vi "what dont like.vi"() -> ()   [LabVIEW 2017]
uses:
  what.ctl
  <vilib>/myRIO/Instrument Drivers/Onboard IO/DIO/typedefs/DIO Reference.ctl
  <vilib>/myRIO/Common/Instrument Driver Framework/Utilities/typedefs/myRIO Generic Hardware Reference.ctl
  <vilib>/myRIO/Common/Instrument Driver Framework/Utilities/typedefs/Hardware Version Enum.ctl
  <vilib>/myRIO/Common/Instrument Driver Framework/Utilities/typedefs/myRIO v1.0 Reference.ctl
  <vilib>/myRIO/Common/Instrument Driver Framework/Utilities/typedefs/Generic FPGA Reference.ctl
  <vilib>/myRIO/Common/Instrument Driver Framework/myRIO v1.0/DIO/typedefs/DIO Channels List.ctl
  <vilib>/myRIO/Common/Instrument Driver Framework/myRIO v1.0/DIO/typedefs/DIO Channels Enum.ctl
  <vilib>/userdefined/High Color/nirio_resource_hc.ctl
  <vilib>/myRIO/Common/Instrument Driver Framework/Utilities/vis/Is FPGA Ref Available.vi
  <vilib>/myRIO/Common/Instrument Driver Framework/myRIO v1.0/DIO/vis/myRIO v1.1 Open DIO.vi
  <vilib>/myRIO/Instrument Drivers/Onboard IO/DIO/vis/Read.vi
  <vilib>/myRIO/Common/Instrument Driver Framework/Utilities/vis/Validate Channels.vi
  <vilib>/myRIO/Common/Instrument Driver Framework/myRIO v1.0/DIO/vis/myRIO v1.0 Reserve DIO.vi
  <vilib>/myRIO/Common/Instrument Driver Framework/myRIO v1.0/Resource Manager/vis/myRIO v1.0 Reserve Channel List.vi
  <vilib>/myRIO/Common/Instrument Driver Framework/myRIO v1.0/DIO/vis/myRIO v1.0 Build MUX Configuration DIO.vi
  <vilib>/myRIO/Common/Instrument Driver Framework/myRIO v1.0/Resource Manager/vis/myRIO v1.0 Reserve Channel.vi
  <vilib>/myRIO/Common/Instrument Driver Framework/myRIO v1.0/Resource Manager/vis/myRIO v1.0 Unreserve Channel.vi
  <vilib>/myRIO/Common/Instrument Driver Framework/myRIO v1.0/Resource Manager/vis/myRIO v1.0 Create Configuration List.vi
  <vilib>/myRIO/Common/Instrument Driver Framework/myRIO v1.0/Resource Manager/vis/myRIO v1.0 Build Mutex Name.vi
  <vilib>/Utility/VariantDataType/GetNumericInfo.vi
  <vilib>/Utility/error.llb/Error Cluster From Error Code.vi
  <vilib>/myRIO/Common/Instrument Driver Framework/myRIO v1.0/myRIO v1.1 Open.vi
  <vilib>/myRIO/Common/Instrument Driver Framework/Utilities/vis/IO Manager.vi
  <vilib>/myRIO/Common/Instrument Driver Framework/Utilities/vis/Configuration Manager.vi
  <vilib>/myRIO/Common/Instrument Driver Framework/myRIO v1.0/Resource Manager/vis/myRIO v1.0 Configure IO.vi
  <vilib>/myRIO/Common/Instrument Driver Framework/myRIO v1.0/myRIO v1.0 Close.vi
  <vilib>/myRIO/Common/Instrument Driver Framework/myRIO v1.0/DIO/vis/myRIO v1.0 Read DIO.vi
  <vilib>/myRIO/Express VI/Onboard IO/DI/DI Express VI.xnode
  <vilib>/myRIO/Instrument Drivers/Onboard IO/DIO/vis/myRIO DIO Open.xnode
  <vilib>/myRIO/Instrument Drivers/Onboard IO/DIO/DIO.lvlib
panel:
  out "index of element":i32
  in  "Stop":bool
  out "Counter Value":dbl
  in  "stop":bool
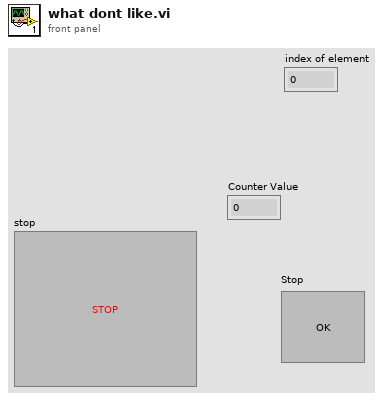
[diagram p1: front panel]
types:
  T1 = typedef "what.ctl" = enum16{"Initialize", "Floor 1", "Floor 2", "Floor 3", "GO!", "Stop!", "Wait for User Input"}
  T2 = typedef "DIO.lvlib/DIO Reference.ctl" = cluster{"myRIO Reference":T3, "DIO Channels List":T7}
  T3 = typedef "myRIO Generic Hardware Reference.ctl" = cluster{"myRIO Model":T4, "myRIO Hardware Reference":T5}
  T4 = typedef "Hardware Version Enum.ctl" = enum16{"Unknown", "myRIO-1900", "myRIO-1950", "roboRIO", "NI ELVIS RIO CM"}
  T5 = typedef "myRIO v1.0 Reference.ctl" = cluster{"Generic FPGA Reference":T6, "Allow multiple opens":bool}
  T6 = typedef "Generic FPGA Reference.ctl" = refnum<k20>
  T7 = typedef "DIO Channels List.ctl" = T8[]
  T8 = typedef "DIO Channels Enum.ctl" = enum16{"Not Connected", "C/DIO0", "C/DIO1", "C/DIO2", "C/DIO3", "C/DIO4", "C/DIO5", "C/DIO6", "C/DIO7", "A/DIO0", "A/DIO1", "A/DIO2", "A/DIO3", "A/DIO4", "A/DIO5", "A/DIO6", "A/DIO7", "A/DIO8", "A/DIO9", "A/DIO10", "A/DIO11", "A/DIO12", "A/DIO13", "A/DIO14", "A/DIO15", "B/DIO0", "B/DIO1", "B/DIO2", "B/DIO3", "B/DIO4", "B/DIO5", "B/DIO6", "B/DIO7", "B/DIO8", "B/DIO9", "B/DIO10", "B/DIO11", "B/DIO12", "B/DIO13", "B/DIO14", "B/DIO15", "LED0", "LED1", "LED2", "LED3", "Button0", "DIO/DIO0", "DIO/DIO1", "DIO/DIO2", "DIO/DIO3", "DIO/DIO4", "DIO/DIO5", "DIO/DIO6", "DIO/DIO7", "DIO/DIO8", "DIO/DIO9", "SPI/CS0", "SPI/CS1", "SPI/CS2", "SPI/CS3", "LED RADIO (Green)", "LED RADIO (Red)", "LED COMM (Green)", "LED COMM (Red)", "LED MODE (Green)", "LED MODE (Red)"}
  T9 = typedef "nirio_resource_hc.ctl" = tag
  T10 = enum16{"off", "flash", "top", "middle", "bottom"}
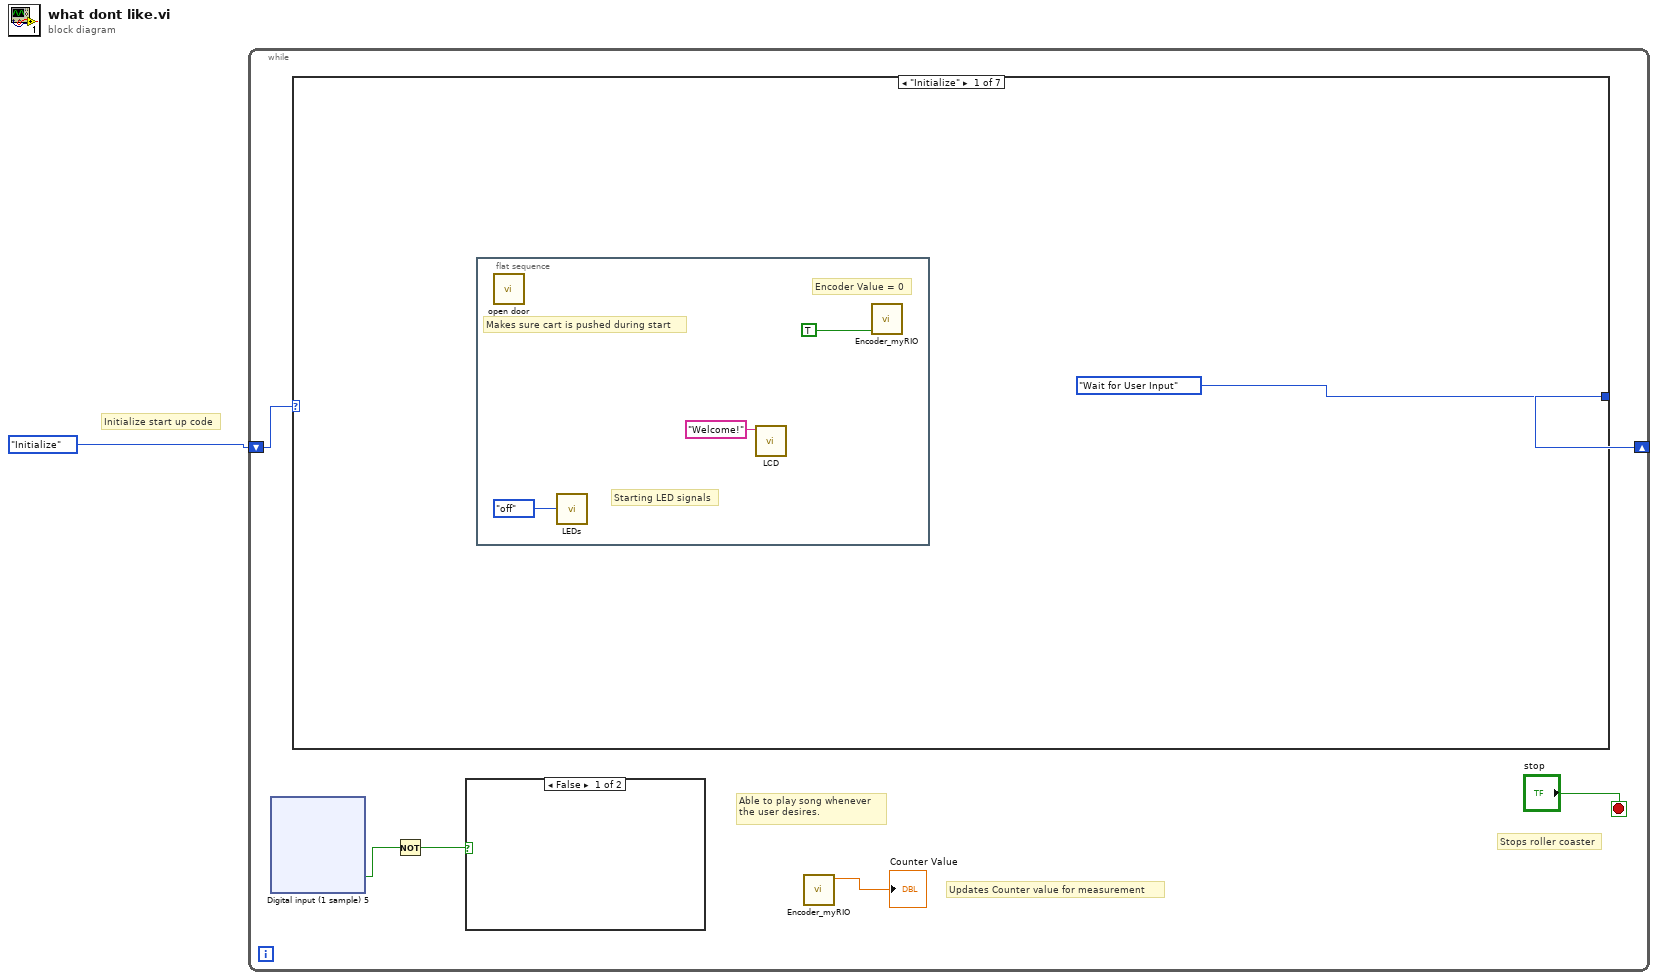
[diagram p0: block diagram]
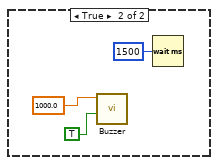
[diagram p2: hidden frame]
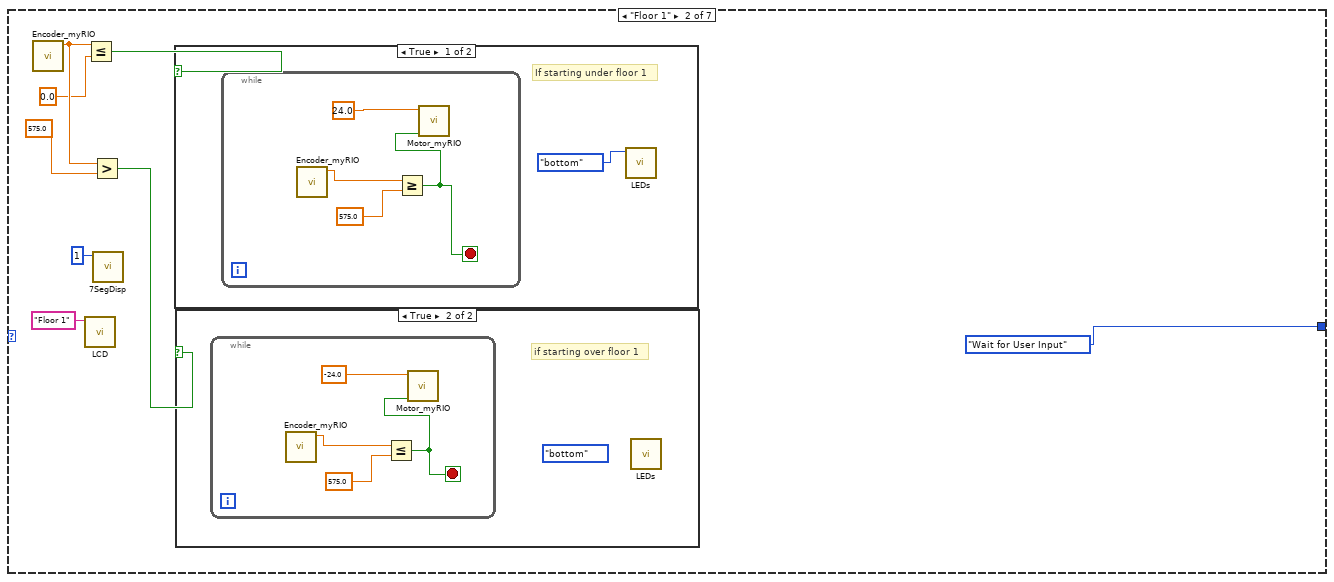
[diagram p3: hidden frame]
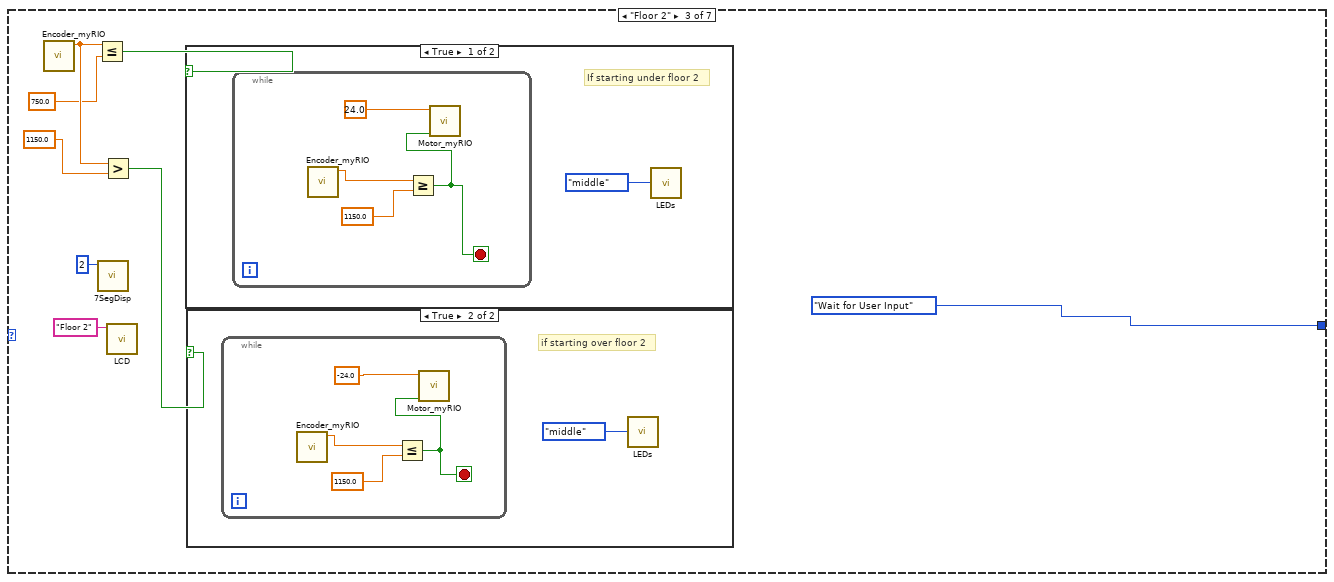
[diagram p6: hidden frame]
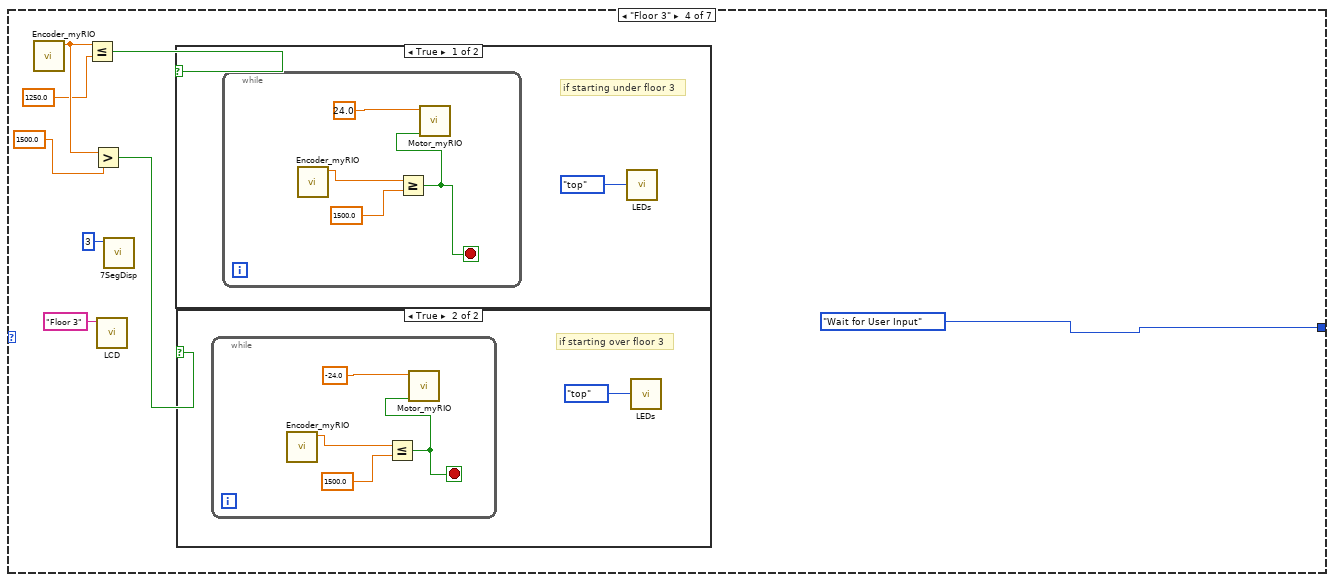
[diagram p9: hidden frame]
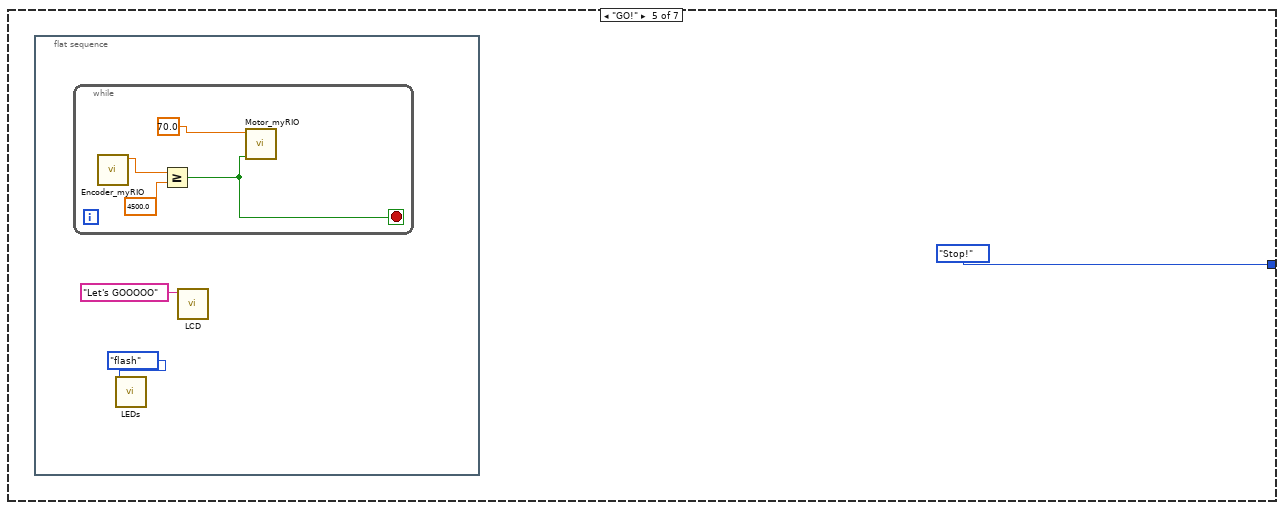
[diagram p12: hidden frame]
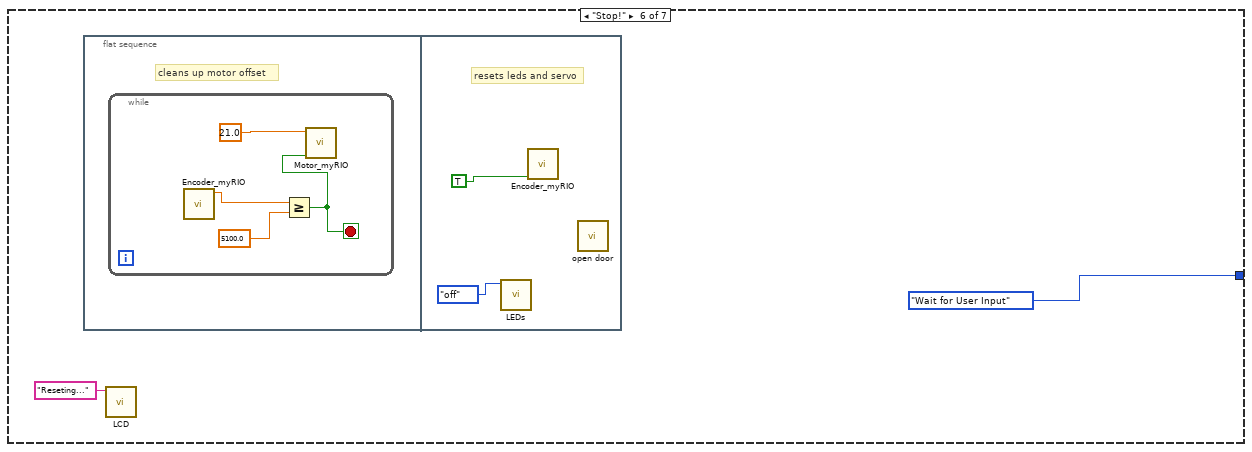
[diagram p13: hidden frame]
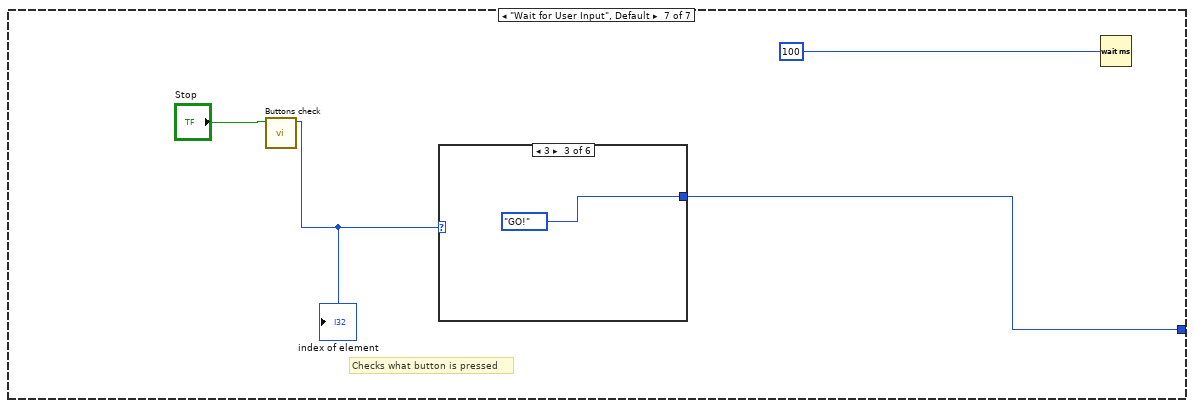
[diagram p14: hidden frame]
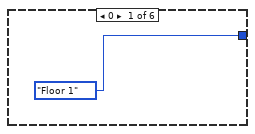
[diagram p15: hidden frame]
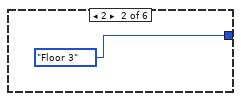
[diagram p16: hidden frame]
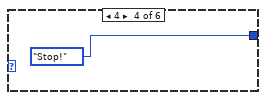
[diagram p17: hidden frame]
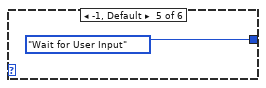
[diagram p18: hidden frame]
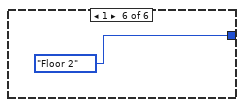
[diagram p19: hidden frame]
diagram:
  # "Initialize start up code"
  n1 = while {
    shift-right: [w7] -> _
    shift-left: what."Initialize" -> [w4]
    stop <- "stop" stop-if-true
    # "Able to play song whenever\nthe user desires."
    # "Stops roller coaster"
    # "Updates Counter value for measurement"
    n2 = xnode "Digital input (1 sample) 5"() -> ("B/DIO14 (Pin 32)"=w2:bool)  [unwired: 1 in, 1 out]
    n3 = case shown="\"Initialize\"" w4 {
      tunnel: [what."Wait for User Input" what."Wait for User Input" what."Wait for User Input" what."Wait for User Input" what."Stop!" what."Wait for User Input" w121] -> w7
      frame "Initialize" {
        n4 = flat-sequence {
          frame #0 {
            # "Starting LED signals"
            # "Makes sure cart is pushed during start"
            # "Encoder Value = 0"
            n5 = call "open door.vi"() -> ()  [unwired: 12 in]
            n6 = call "LEDs.vi"("Enum"=T10."off") -> ()  [unwired: 11 in]
            n7 = call "LCD.vi"("String"="Welcome!") -> ()  [unwired: 11 in]
            n8 = call "Encoder_myRIO.vi"("Reset"=TRUE) -> ()  [unwired: 9 in, 2 out]
          }
        }
      }
      frame "Floor 1" {
        n9 = call "Encoder_myRIO.vi"() -> ("Counter Value"=w54:dbl)  [unwired: 10 in, 1 out]
        n10 = call "LCD.vi"("String"="Floor 1") -> ()  [unwired: 11 in]
        n11 = Less Or Equal?(x=w54, y=0.0) -> (x <= y?=w56:bool)
        n12 = Greater?(x=w54, y=575.0) -> (0:w55:bool)
        n13 = call "7SegDisp.vi"("Input Number"=1) -> ()  [unwired: 11 in]
        n14 = case shown="True" w56 {
          frame True {
            # "If starting under floor 1"
            n15 = while {
              stop <- w59 stop-if-true
              n16 = call "Encoder_myRIO.vi"() -> ("Counter Value"=w62:dbl)  [unwired: 10 in, 1 out]
              n17 = Greater Or Equal?(x=w62, y=575.0) -> (x >= y?=w59:bool)
              n18 = call "Motor_myRIO.vi"("Stop VI"=w59, "Duty Cycle (-100 to +100)"=24.0) -> ()  [unwired: 10 in]
            }
            n19 = call "LEDs.vi"("Enum"=T10."bottom") -> ()  [unwired: 11 in]
          }
          frame False {
          }
        }
        n20 = case shown="True" w55 {
          frame False {
          }
          frame True {
            (unwired) T10."bottom" ("Enum")
            # "if starting over floor 1"
            n21 = while {
              stop <- w63 stop-if-true
              n22 = call "Encoder_myRIO.vi"() -> ("Counter Value"=w66:dbl)  [unwired: 10 in, 1 out]
              n23 = Less Or Equal?(x=w66, y=575.0) -> (x <= y?=w63:bool)
              n24 = call "Motor_myRIO.vi"("Stop VI"=w63, "Duty Cycle (-100 to +100)"=-24.0) -> ()  [unwired: 10 in]
            }
            n25 = call "LEDs.vi"() -> ()  [unwired: 12 in]
          }
        }
      }
      frame "Floor 2" {
        n26 = call "Encoder_myRIO.vi"() -> ("Counter Value"=w71:dbl)  [unwired: 10 in, 1 out]
        n27 = Less Or Equal?(x=w71, y=750.0) -> (x <= y?=w73:bool)
        n28 = call "7SegDisp.vi"("Input Number"=2) -> ()  [unwired: 11 in]
        n29 = Greater?(x=w71, y=1150.0) -> (0:w72:bool)
        n30 = call "LCD.vi"("String"="Floor 2") -> ()  [unwired: 11 in]
        n31 = case shown="True" w73 {
          frame True {
            # "If starting under floor 2"
            n32 = while {
              stop <- w76 stop-if-true
              n33 = call "Encoder_myRIO.vi"() -> ("Counter Value"=w79:dbl)  [unwired: 10 in, 1 out]
              n34 = Greater Or Equal?(x=w79, y=1150.0) -> (x >= y?=w76:bool)
              n35 = call "Motor_myRIO.vi"("Stop VI"=w76, "Duty Cycle (-100 to +100)"=24.0) -> ()  [unwired: 10 in]
            }
            n36 = call "LEDs.vi"("Enum"=T10."middle") -> ()  [unwired: 11 in]
          }
          frame False {
          }
        }
        n37 = case shown="True" w72 {
          frame False {
          }
          frame True {
            # "if starting over floor 2"
            n38 = while {
              stop <- w81 stop-if-true
              n39 = call "Encoder_myRIO.vi"() -> ("Counter Value"=w84:dbl)  [unwired: 10 in, 1 out]
              n40 = Less Or Equal?(x=w84, y=1150.0) -> (x <= y?=w81:bool)
              n41 = call "Motor_myRIO.vi"("Stop VI"=w81, "Duty Cycle (-100 to +100)"=-24.0) -> ()  [unwired: 10 in]
            }
            n42 = call "LEDs.vi"("Enum"=T10."middle") -> ()  [unwired: 11 in]
          }
        }
      }
      frame "Floor 3" {
        n43 = call "Encoder_myRIO.vi"() -> ("Counter Value"=w89:dbl)  [unwired: 10 in, 1 out]
        n44 = Less Or Equal?(x=w89, y=1250.0) -> (x <= y?=w91:bool)
        n45 = Greater?(x=w89, y=1500.0) -> (0:w90:bool)
        n46 = call "LCD.vi"("String"="Floor 3") -> ()  [unwired: 11 in]
        n47 = call "7SegDisp.vi"("Input Number"=3) -> ()  [unwired: 11 in]
        n48 = case shown="True" w91 {
          frame True {
            # "if starting under floor 3"
            n49 = while {
              stop <- w94 stop-if-true
              n50 = call "Encoder_myRIO.vi"() -> ("Counter Value"=w97:dbl)  [unwired: 10 in, 1 out]
              n51 = Greater Or Equal?(x=w97, y=1500.0) -> (x >= y?=w94:bool)
              n52 = call "Motor_myRIO.vi"("Stop VI"=w94, "Duty Cycle (-100 to +100)"=24.0) -> ()  [unwired: 10 in]
            }
            n53 = call "LEDs.vi"("Enum"=T10."top") -> ()  [unwired: 11 in]
          }
          frame False {
          }
        }
        n54 = case shown="True" w90 {
          frame False {
          }
          frame True {
            # "if starting over floor 3"
            n55 = while {
              stop <- w100 stop-if-true
              n56 = call "Encoder_myRIO.vi"() -> ("Counter Value"=w102:dbl)  [unwired: 10 in, 1 out]
              n57 = Less Or Equal?(x=w102, y=1500.0) -> (x <= y?=w100:bool)
              n58 = call "Motor_myRIO.vi"("Stop VI"=w100, "Duty Cycle (-100 to +100)"=-24.0) -> ()  [unwired: 10 in]
            }
            n59 = call "LEDs.vi"("Enum"=T10."top") -> ()  [unwired: 11 in]
          }
        }
      }
      frame "GO!" {
        n60 = flat-sequence {
          frame #0 {
            n61 = while {
              stop <- w106 stop-if-true
              n62 = call "Encoder_myRIO.vi"() -> ("Counter Value"=w108:dbl)  [unwired: 10 in, 1 out]
              n63 = Greater Or Equal?(x=w108, y=4500.0) -> (x >= y?=w106:bool)
              n64 = call "Motor_myRIO.vi"("Stop VI"=w106, "Duty Cycle (-100 to +100)"=70.0) -> ()  [unwired: 10 in]
            }
            n65 = call "LEDs.vi"("Enum"=T10."flash") -> ()  [unwired: 11 in]
            n66 = call "LCD.vi"("String"="Let's GOOOOO") -> ()  [unwired: 11 in]
          }
        }
      }
      frame "Stop!" {
        n67 = flat-sequence {
          frame #0 {
            # "cleans up motor offset"
            n68 = while {
              stop <- w112 stop-if-true
              n69 = call "Encoder_myRIO.vi"() -> ("Counter Value"=w115:dbl)  [unwired: 10 in, 1 out]
              n70 = Greater Or Equal?(x=w115, y=5100.0) -> (x >= y?=w112:bool)
              n71 = call "Motor_myRIO.vi"("Stop VI"=w112, "Duty Cycle (-100 to +100)"=21.0) -> ()  [unwired: 10 in]
            }
          }
          frame #1 {
            # "resets leds and servo"
            n72 = call "LEDs.vi"("Enum"=T10."off") -> ()  [unwired: 11 in]
            n73 = call "Encoder_myRIO.vi"("Reset"=TRUE) -> ()  [unwired: 9 in, 2 out]
            n74 = call "open door.vi"() -> ()  [unwired: 12 in]
          }
        }
        n75 = call "LCD.vi"("String"="Reseting...") -> ()  [unwired: 11 in]
      }
      frame "Wait for User Input", Default {
        # "Checks what button is pressed"
        n76 = call "Buttons check.vi"("Abort"="Stop") -> ("index of element"=w119:i32)  [unwired: 10 in]
        "index of element" <- w119
        n77 = case shown="3" w119 {
          tunnel: [what."Floor 1" what."Floor 3" what."GO!" what."Stop!" what."Wait for User Input" what."Floor 2"] -> w121
          frame 0 {
          }
          frame 2 {
          }
          frame 3 {
          }
          frame 4 {
          }
          frame -1, Default {
          }
          frame 1 {
          }
        }
        n78 = Wait (ms)(milliseconds to wait=u32 100) -> ()  [unwired: 1 out]
      }
    }
    n79 = Not(x=w2) -> (.not. x?=w3:bool)
    n80 = case shown="False" w3 {
      frame False {
      }
      frame True {
        n81 = call "Buzzer.vi"("stop"=TRUE, "frequency [Hz]"=1000.0) -> ()  [unwired: 10 in]
        n82 = Wait (ms)(milliseconds to wait=u32 1500) -> ()  [unwired: 1 out]
      }
    }
    n83 = call "Encoder_myRIO.vi"() -> ("Counter Value"=→"Counter Value":dbl)  [unwired: 10 in, 1 out]
  }
